vi "Auto Vertical Conveyor.vi"(9 "seconds":dbl) -> (1 "stop":bool)   [LabVIEW 2019]
uses:
  Robot Global Data.vi
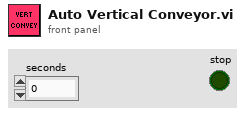
[diagram p1: front panel]
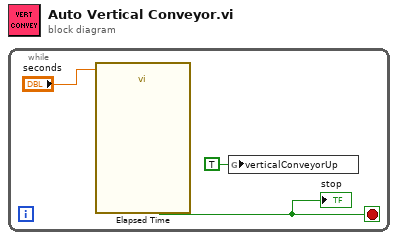
[diagram p0: block diagram]
diagram:
  n1 = while {
    stop <- w1 stop-if-true
    n2 = call "Elapsed Time"("Time Target (s)"="seconds") -> ("Time has Elapsed"=w1:bool)  [unwired: 11 in, 7 out]
    "stop" <- w1
    n3 = global write "Robot Global Data.vi" "verticalConveyorUp"(TRUE ("verticalConveyorUp")) -> ()
  }
